vi "Move Axes to Positions.vi"(7 "error in (no error)":errorcluster, 8 "Array of positions [internal units]":dbl[](array[numeric]) format="%#_8f", 9 "Array of axes":T1[](array[typedef]), 10 "VISA in":refnum<visa-resource-name>) -> (0 "error out":errorcluster, 3 "VISA out":refnum<visa-resource-name>)   [LabVIEW 2017, in "Drivers.lvlib" / "ASI TG-1000.lvlib"]
doc: "Tells the ASI controller to move the specified axes to the corresponding specified positions; the equivalent of using the MOVE command with multiple arguments. Note that it performs no checking to see if the move completes successfully."
uses:
  ASI TG-1000.lvlib
  Utility/Axis Name.ctl
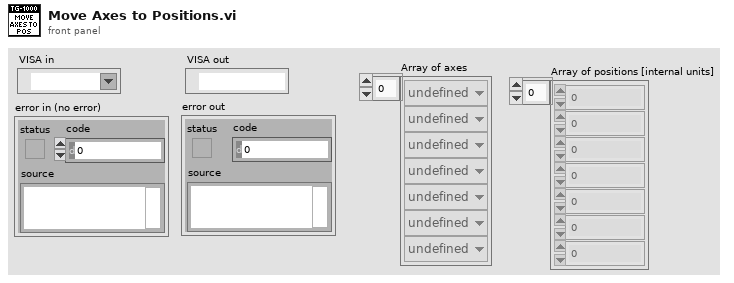
[diagram p1: front panel]
types:
  T1 = typedef "Drivers.lvlib/ASI TG-1000.lvlib/Axis Name.ctl" = enum8{"undefined", "A", "B", "C", "D", "E", "F", "G", "H", "I", "J", "K", "L", "M", "N", "O", "P", "Q", "R", "S", "T", "U", "V", "W", "X", "Y", "Z"}
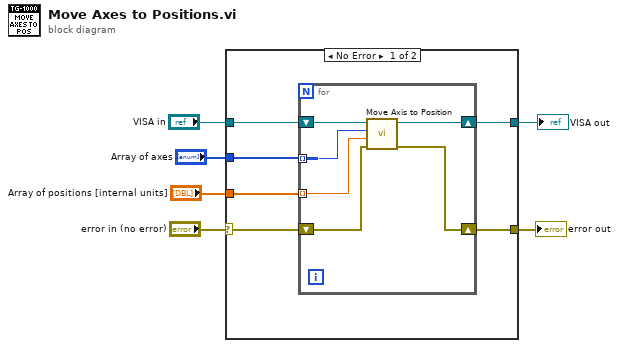
[diagram p0: block diagram]
diagram:
  n1 = case shown="No Error" "error in (no error)" {
    selector: "error in (no error)" -> [w7 w19]
    tunnel: "Array of positions [internal units]" -> [w12 _]
    tunnel: "Array of axes" -> [w11 _]
    tunnel: "VISA in" -> [w10 w20]
    tunnel: [w9 w20] -> w3
    tunnel: [w8 w19] -> w2
    frame No Error {
      n2 = for {
        tunnel: w11 -> [w17] mode=indexing
        tunnel: w12 -> [w16] mode=indexing
        shift-right: [w15] -> w9
        shift-left: w10 -> [w18]
        shift-right: [w14] -> w8
        shift-left: w7 -> [w13]
        n3 = call "Move Axis to Position.vi"("error in (no error)"=w13, "Position [internal units]"=w16, "Axis"=w17, "VISA in"=w18) -> ("error out"=w14:errorcluster, "VISA out"=w15:refnum<visa-resource-name>)  [unwired: 5 in]
      }
    }
    frame Error {
    }
  }
  "VISA out" <- w3
  "error out" <- w2
